vi "Set Main FPGA Chassis Slots Programming Mode.vi"(8 "error in (no error)":errorcluster, 10 "serverName in":string="10.0.18.244", 11 "Item Ref in":T1 format="%.0x") -> (0 "error out":errorcluster, 2 "serverName out":string="10.0.18.244", 3 "Item Ref out":T1 format="%.0x")   [LabVIEW 2026, in "SEECD System Explorer.lvlib"]
doc: "Goal of this VI is to set the slot \"Programming Mode\" property for recent cRIO chassis (NI-904x, NI-905x,...) in accordance to control \"FPGA / Scan interface mode\" control of Target main Configuration page, in \"Othe Settings\" section.\n------------------------------------------------------------------------------------------------------\nIMPLEMENTATION\nThis VI checks the value of property \"FPGA / Scan interface mode\" of Target Configuration Page."
uses:
  SEECD System Explorer.lvlib
  <vilib>/NI VeriStand/Custom Device Tools/Custom Device Utility Library/Custom Device Utility Library.lvlib
  <vilib>/NI VeriStand/Custom Device Offline API/Custom Device Offline API.lvlib
  NationalInstruments.VeriStand.SystemDefinitionAPI
  C:/Users/Administrator/Desktop/Jatin/All DNC DLLs/NationalInstruments.VeriStand.SystemDefinitionAPI.dll
  Jatin/All DNC DLLs/NationalInstruments.VeriStand.SystemDefinitionAPI.dll
  <vilib>/NI VeriStand/Custom Device API/Custom Device Item Ref.ctl
  <vilib>/NI VeriStand/Custom Device API/Custom Device API.lvlib
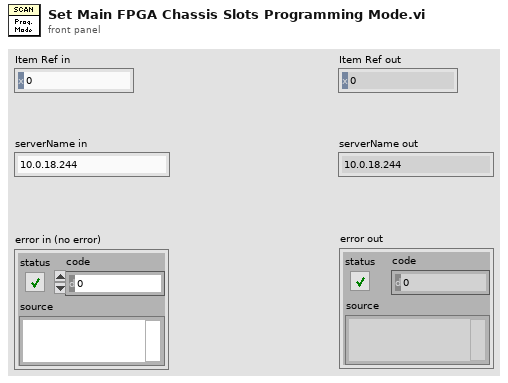
[diagram p1: front panel]
types:
  T1 = typedef "Custom Device API.lvlib/Custom Device Item Ref.ctl" = u64
  T2 = typedef "SEECD System Explorer.lvlib/Slot Programming Mode.ctl" = enum16{"Don't Modify", "Scan Engine", "LabVIEW FPGA", "NI-DAQmx"}
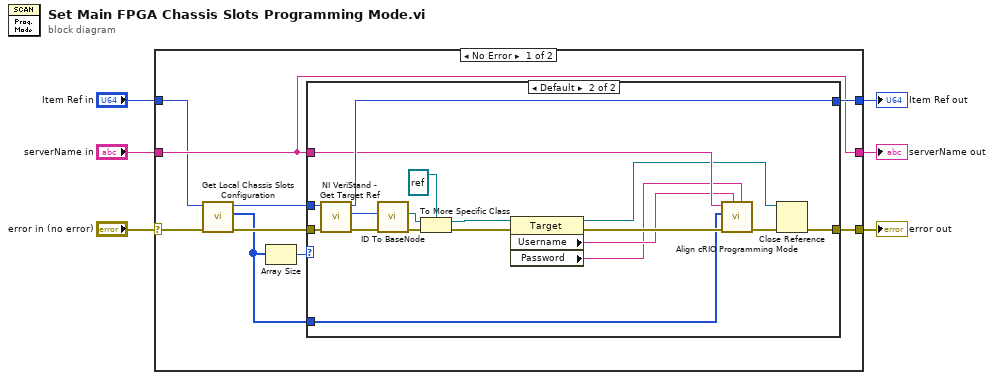
[diagram p0: block diagram]
diagram:
  n1 = case shown="No Error" "error in (no error)" {
    selector: "error in (no error)" -> [w11 w38]
    tunnel: [w14 w38] -> w5
    tunnel: "Item Ref in" -> [w12 w37]
    tunnel: [w15 w37] -> w3
    tunnel: "serverName in" -> [w13 w36]
    tunnel: [w13 w36] -> w1
    frame No Error {
      n2 = call "Get Local Chassis Slots Configuration.vi"("error in (no error)"=w11, "Item Ref in"=w12) -> ("error out"=w9:errorcluster, "Slots Configuration"=w7:T2[], "Item Ref out"=w10:T1)  [unwired: 7 in]
      n3 = Array Size(array=w7) -> (size(s)=w8:i32)
      n4 = case shown="Default" w8 {
        tunnel: [w17 w31] -> w15
        tunnel: [w16 w27] -> w14
        tunnel: w13 -> [_ w25]
        tunnel: w10 -> [w17 w23]
        tunnel: w9 -> [w16 w22]
        tunnel: w7 -> [_ w18]
        frame 0 {
          # "No modules configured in Local Chassis in Sysdef."
        }
        frame Default {
          n5 = call <vilib>:"NI VeriStand - Get Target Ref.vi"("error in"=w22, "Item Ref in"=w23) -> ("error out"=w30:errorcluster, "Target Ref"=w35:T1, "Item Ref out"=w31:T1)  [unwired: 6 in, 1 out]
          n6 = call <vilib>:"ID To BaseNode.vi"("error in (no error)"=w30, "ID in"=w35) -> ("error out"=w29:errorcluster, "BaseNode"=w33:refnum<k24>)  [unwired: 7 in, 1 out]
          n7 = To More Specific Class(target class=refnum<k39> refnum, reference=w33, error in=w29) -> (specific class reference=w34:refnum<k39>, error out=w28:errorcluster)
          n8 = property class="Target"(reference=w34, error in=w28) -> (reference out=w21:refnum<k39>, error out=w24:errorcluster, "Username"=w20:string, "Password"=w19:string)
          n9 = call "Align cRIO Programming Mode.vi"("Password"=w19, "User Name"=w20, "error in (no error)"=w24, "Slots Configuration"=w18, "Target (localhost)"=w25) -> ("error out"=w26:errorcluster)  [unwired: 6 in]
          n10 = Close Reference(reference=w21, error in (no error)=w26) -> (error out=w27:errorcluster)
        }
      }
    }
    frame Error {
    }
  }
  "error out" <- w5
  "Item Ref out" <- w3
  "serverName out" <- w1
